vi "Is PMT ON.vi"(1 "Channel":T1) -> (0 "PMT is ON":bool)   [LabVIEW 2017]
uses:
  Typedefs/Channel Selector.ctl
panel:
  # "SUBROUTINE VI"
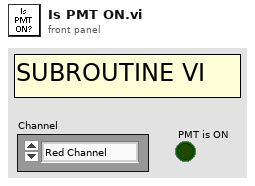
[diagram p1: front panel]
types:
  T1 = typedef "Channel Selector.ctl" = enum16{"Red Channel", "Green Channel", "Blended"}
  T2 = typedef "AOL_Globals.ctl" = cluster{"Imaging Protocol":T3, "Number of POI":u16, "Number of Miniscans":u16, "Number of Trials":u16, "Number of Cycles ":u64, "# Averaged Frames":u16, "Laser power (%)":u8, "Pockels":dbl, "Acquisition Length (sec)":dbl, "Fill time (us)":dbl, "POI Dwell time (us)":dbl, "Miniscan Dwell time per pixel (us)":dbl, "PMT 1":dbl, "PMT 2":dbl, "Back Apperture":dbl, "Frame Size":T4, "Center Frequency":dbl, "Field of View":dbl, "DwellTime (us)":dbl, "Wavelength (nm)":dbl, "Zoom":dbl, "AOL Z":dbl, "AOL Mode":T5, "GridXY":dbl, "GridZ":dbl, "TriggerPeriod (sec)":dbl, "Number of Pixels in Miniscan":u16, "Experiment folder path":path, "X centre":dbl, "Y centre":dbl, "Angle (degrees)":dbl, "Plane Mode":T6, "Threshold":u16[], "Regenerate Chirps":bool, "Rectangle ROI length (pixels)":u16, "Rectangle ROI height (pixels)":u16, "AOD fill":u16, "StartupDelay":i32, "Samples Wait after Trigger":u16, "Slip Cycle":u32, "Add Cycle":bool}
  T3 = typedef "Imaging Protocols enum.ctl" = enum16{"AOL Z-Stack", "Motor Z Stack", "Functional Acquisition", "Single Plane Acquisition", "Volume Acquisition", "Live Imaging", "Live Plane Imaging", "Live Volume Imaging"}
  T4 = typedef "Frame Size.ctl" = u16
  T5 = typedef "AOL modes.ctl" = enum16{"Raster", "Structural", "Pointing", "Mini Scan", "Alignment"}
  T6 = typedef "Plane Mode.ctl" = u16
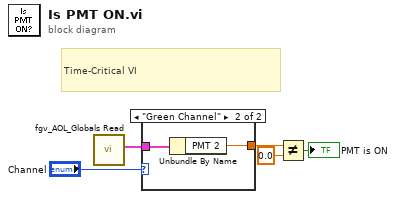
[diagram p0: block diagram]
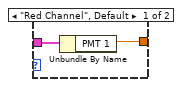
[diagram p2: hidden frame]
diagram:
  # "Time-Critical VI"
  n1 = call "fgv_AOL_Globals Read.vi"() -> ("AOL_Globals"=w3:T2)  [unwired: 9 in, 2 out]
  n2 = case shown="\"Green Channel\"" "Channel" {
    tunnel: w3 -> [w7 w9]
    tunnel: [w6 w8] -> w2
    frame "Red Channel", Default {
      n3 = Unbundle By Name(w7) -> ("PMT 1"=w6:dbl)
    }
    frame "Green Channel" {
      n4 = Unbundle By Name(w9) -> ("PMT 2"=w8:dbl)
    }
  }
  n5 = Not Equal?(x=w2, y=0.0) -> (x != y?=→"PMT is ON":bool)
